vi "Run Measure And Log Slide Show.vi"() -> ()   [LabVIEW 2019]
doc: "View a storyboard of the top-down development of a simple Measure and Log application."
panel:
  in  "Exit":bool
  in  "Next":bool
  in  "Previous":bool
  out "Level of Abstraction":i32(slide) min=0 max=6 step=1 scale=0.0..7.0
  # "Measure and Log Storyboard"
  # "high"
  # "low"
  # "Overview: Running this VI will show you a sequence of VIs demonstrating the entire software engineering process of a top-down design for a system that does some data acquisition and logging. It starts with a high level diagram and then refines the design, gradually adding functional details."
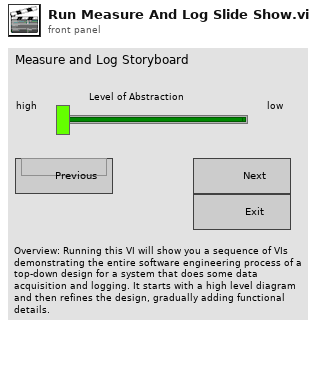
[diagram p1: front panel]
types:
  T1 = typedef "LVRectTypeDef.ctl" = cluster{"Left":i16, "Top":i16, "Right":i16, "Bottom":i16}
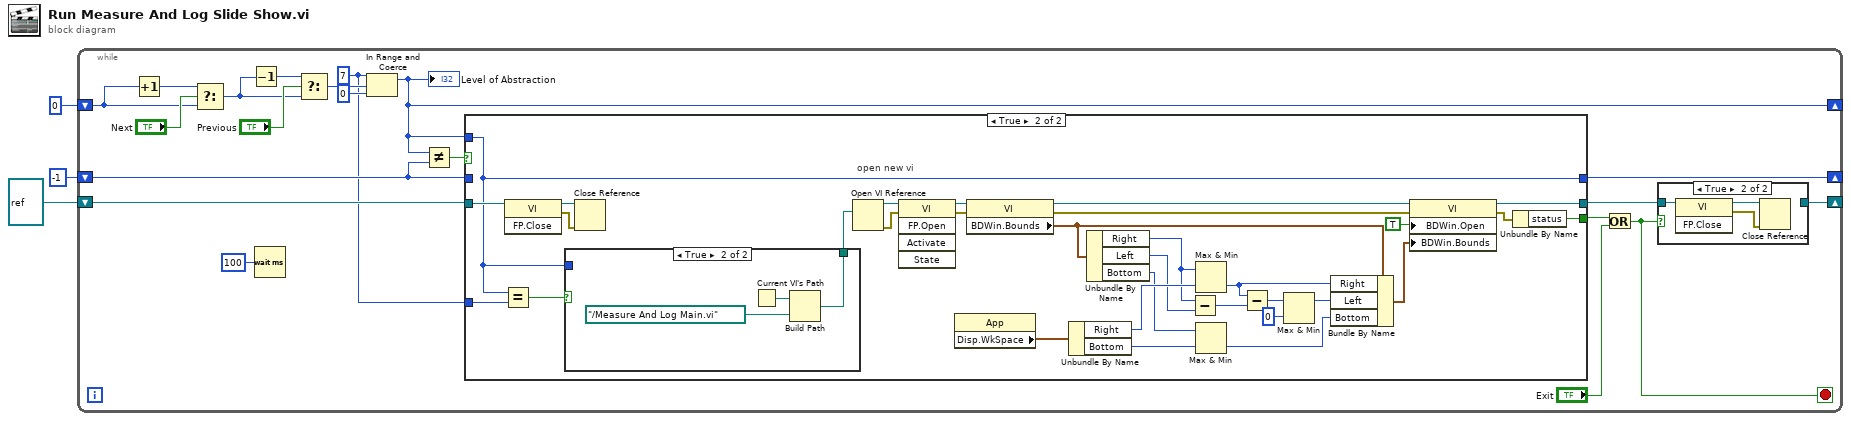
[diagram p0: block diagram]
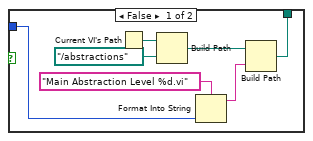
[diagram p3: hidden frame]
diagram:
  n1 = while {
    shift-right: [w11] -> _
    shift-left: 0 -> [w17]
    shift-right: [w13] -> _
    shift-left: -1 -> [w12]
    shift-right: [w6] -> _
    shift-left: refnum<vi> refnum ("vi reference") -> [w10]
    stop <- w8 stop-if-true
    w4 = 7 ("upper limit")
    n2 = Increment(x=w17) -> (x+1=w21:i32)
    n3 = Select(t=w21, s="Next", f=w17) -> (s? t:f=w19:i32)
    n4 = Decrement(x=w19) -> (x-1=w18:i32)
    n5 = Wait (ms)(milliseconds to wait=u32 100) -> ()  [unwired: 1 out]
    n6 = Select(t=w18, s="Previous", f=w19) -> (s? t:f=w16:i32)
    n7 = In Range and Coerce(upper limit=w4, x=w16, lower limit=0) -> (coerced(x)=w11:i32)  [unwired: 1 out]
    "Level of Abstraction" <- w11
    n8 = Not Equal?(x=w11, y=w12) -> (x != y?=w15:bool)
    n9 = case shown="True" w15 {
      tunnel: [w25 w29] -> w13
      tunnel: w11 -> [_ w29]
      tunnel: w12 -> [w25 _]
      tunnel: [w24 w49] -> w7
      tunnel: w10 -> [w24 w55]
      tunnel: [_ w51] -> w9
      tunnel: w4 -> [_ w28]
      frame False {
      }
      frame True {
        # "open new vi"
        n10 = Equal?(x=w29, y=w28) -> (x = y?=w27:bool)
        n11 = invoke class="VI" method="FP.Close"(reference=w55) -> (reference out=w53:refnum<vi>, error out=w54:errorcluster)  [unwired: 2 in, 1 out]
        n12 = case shown="True" w27 {
          tunnel: w29 -> [w62 _]
          tunnel: [w57 w64] -> w26
          frame False {
            n13 = Current VI's Path() -> (path=w60:path)
            n14 = Build Path(base path=w60, name or relative path=path "../abstractions") -> (appended path=w59:path)
            n15 = Format Into String(format string="Main Abstraction Level %d.vi", w62) -> (resulting string=w58:string)  [unwired: 2 in, 1 out]
            n16 = Build Path(base path=w59, name or relative path=w58) -> (appended path=w57:path)
          }
          frame True {
            n17 = Current VI's Path() -> (path=w65:path)
            n18 = Build Path(base path=w65, name or relative path=path "../Measure And Log Main.vi") -> (appended path=w64:path)
          }
        }
        n19 = Close Reference(reference=w53, error in (no error)=w54) -> ()  [unwired: 1 out]
        n20 = Open VI Reference(vi path=w26) -> (vi reference=w56:refnum<vi>, error out=w52:errorcluster)  [unwired: 5 in]
        n21 = invoke class="VI" method="FP.Open"(reference=w56, error in=w52) -> (reference out=w33:refnum<vi>, error out=w32:errorcluster)  [unwired: 3 in, 3 out]
        n22 = property class="App"() -> ("Disp.WkSpace"=w47:T1)  [unwired: 2 in, 2 out]
        n23 = property class="VI"(reference=w33, error in=w32) -> (reference out=w30:refnum<vi>, error out=w31:errorcluster, "BDWin.Bounds"=w45:T1)
        n24 = Unbundle By Name(w47) -> ("Right"=w44:i16, "Bottom"=w35:i16)
        n25 = Unbundle By Name(w45) -> ("Right"=w43:i16, "Left"=w42:i16, "Bottom"=w36:i16)
        n26 = Subtract(x=w43, y=w42) -> (x-y=w40:i16)
        n27 = Max & Min(x=w43, y=w44) -> (min(x,y)=w41:i16)  [unwired: 1 out]
        n28 = Max & Min(x=w36, y=w35) -> (min(x,y)=w34:i16)  [unwired: 1 out]
        n29 = Subtract(x=w41, y=w40) -> (x-y=w39:i16)
        n30 = Max & Min(x=w39, y=i16 0) -> (max(x,y)=w38:i16)  [unwired: 1 out]
        n31 = Bundle By Name(cluster=w45, "Right"=w41, "Left"=w38, "Bottom"=w34) -> (w46:T1)
        n32 = property class="VI"(reference=w30, error in=w31, "BDWin.Open"=TRUE ("Block Diagram Window:Open"), "BDWin.Bounds"=w46) -> (reference out=w49:refnum<vi>, error out=w48:errorcluster)
        n33 = Unbundle By Name(w48) -> ("status"=w51:bool)
      }
    }
    n34 = Or(x=w9, y="Exit") -> (x .or. y?=w8:bool)
    n35 = case shown="True" w8 {
      tunnel: w7 -> [w67 w68]
      tunnel: [w67 _] -> w6
      frame False {
      }
      frame True {
        n36 = invoke class="VI" method="FP.Close"(reference=w68) -> (reference out=w70:refnum<vi>, error out=w69:errorcluster)  [unwired: 2 in, 1 out]
        n37 = Close Reference(reference=w70, error in (no error)=w69) -> ()  [unwired: 1 out]
      }
    }
  }
